vi "Edgertronic-get_storage_info.vi"(3 "error in (no error)":errorcluster, 5 "URL":string="192.168.1.101") -> (0 "error out":errorcluster, 1 "Storage Info:":T1={"Connection Information:"="", "Available Space"="20140911165611", "Mount Point"="20140911165611", "Storage Size"="20140911165611"}, 2 "Storage Status":cluster{"Storage Status":u8, "String":string} {"Storage Status" scale=0.0..100.0})   [LabVIEW 2015]
doc: "This VI returns storage device information."
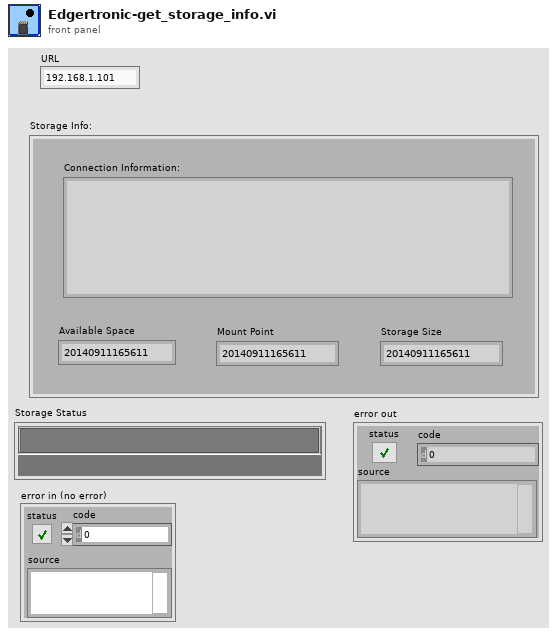
[diagram p1: front panel]
types:
  T1 = cluster{"Connection Information:":string, "Available Space":string, "Mount Point":string, "Storage Size":string}
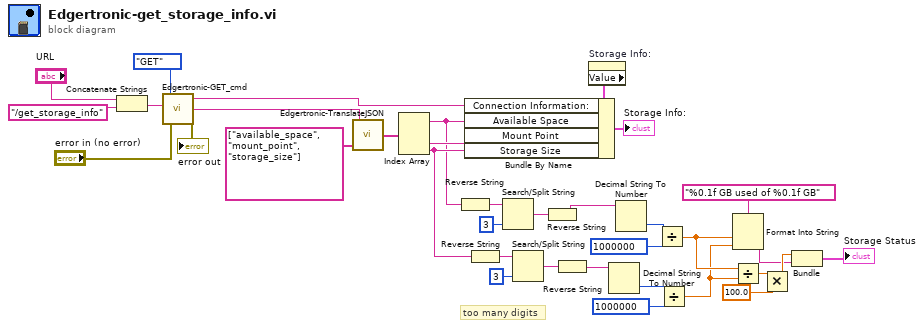
[diagram p0: block diagram]
diagram:
  # "too many digits"
  n1 = Concatenate Strings("URL", "/get_storage_info" ("GET Cmd")) -> (w2:string)
  n2 = call "Edgertronic-GET_cmd.vi"("error in (no error)"="error in (no error)", "URL"=w2, "Type"=enum16{"GET", "POST"}."GET") -> ("error out"=→"error out":errorcluster, "data"=w30:string, "Connection Info"=w33:string)  [unwired: 1 in]
  n3 = call "Edgertronic-TranslateJSON.vi"("Commands"=string[] ["available_space", "mount_point", "storage_size"], "data"=w30) -> ("Values"=w31:string[])  [unwired: 3 in]
  n4 = Index Array(array=w31) -> (element #1=w6:string, element #2=w29:string, element #3=w15:string)  [unwired: 3 in]
  n5 = Reverse String(1:w6) -> (0:w7:string)
  n6 = Reverse String(1:w15) -> (0:w14:string)
  n7 = Search/Split String(string=w7, offset (0)=3) -> (match + rest of string=w9:string)  [unwired: 1 in, 2 out]
  n8 = Search/Split String(string=w14, offset (0)=3) -> (match + rest of string=w12:string)  [unwired: 1 in, 2 out]
  n9 = Reverse String(1:w9) -> (0:w5:string)
  n10 = Reverse String(1:w12) -> (0:w11:string)
  n11 = property on="Storage Info:" class="Clust (strict)"() -> ("Value"=w32:T1)  [unwired: 2 in, 2 out]
  n12 = Bundle By Name(cluster=w32, "Connection Information:"=w33, "Available Space"=w6, "Mount Point"=w29, "Storage Size"=w15) -> (→"Storage Info:":T1)
  n13 = Decimal String To Number(string=w11) -> (number=w10:i32)  [unwired: 2 in, 1 out]
  n14 = Decimal String To Number(string=w5) -> (number=w27:i32)  [unwired: 2 in, 1 out]
  n15 = Divide(x=w27, y=1000000) -> (x/y=w23:dbl)
  n16 = Divide(x=w10, y=1000000) -> (x/y=w22:dbl)
  n17 = Format Into String(format string="%0.1f GB used of %0.1f GB", w23, w22) -> (resulting string=w18:string)  [unwired: 2 in, 1 out]
  n18 = Divide(x=w23, y=w22) -> (x/y=w21:dbl)
  n19 = Multiply(x=w21, y=100.0) -> (x*y=w19:dbl)
  n20 = Bundle(w19, w18) -> (→"Storage Status":cluster{dbl, string})  [unwired: 1 in]
